vi "TaskFor_P3AT_Co_Boundary_Message.vi"(8 "error in (no error)":errorcluster caption="错误输入（无错误）", 10 "P3AT_Boundary":T1 {"max_rot" scale=0.0..1.0; "max_vel" scale=0.0..1.0}, 11 "Remote Endpoint P3AT输入":refnum<class "RemoteP3AT.lvclass">) -> (0 "error out":errorcluster caption="错误输出", 3 "Remote Endpoint P3AT输出":refnum<class "RemoteP3AT.lvclass">)   [LabVIEW 2014]
uses:
  RemoteP3AT.lvclass
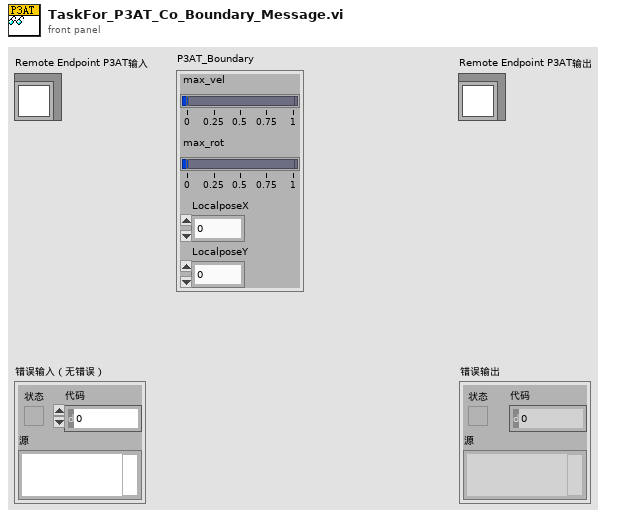
[diagram p1: front panel]
types:
  T1 = cluster{"max_vel":dbl, "max_rot":dbl, "LocalposeX":i32, "LocalposeY":i32}
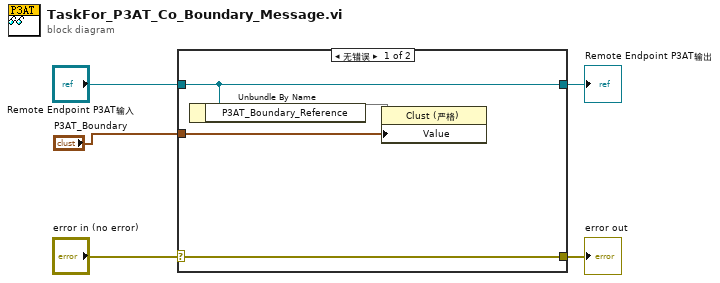
[diagram p0: block diagram]
diagram:
  n1 = case shown="无错误" "error in (no error)" {
    selector: "error in (no error)" -> [w9 w10]
    tunnel: [w9 w10] -> w4
    tunnel: [w8 w11] -> w2
    tunnel: "Remote Endpoint P3AT输入" -> [w8 w11]
    tunnel: "P3AT_Boundary" -> [w6 _]
    frame No Error {
      n2 = Unbundle By Name(w8) -> ("P3AT_Boundary_Reference"=w7)
      n3 = property class="Clust (严格)"(reference=w7, "Value"=w6) -> ()  [unwired: 1 in, 2 out]
    }
    frame Error {
    }
  }
  "error out" <- w4
  "Remote Endpoint P3AT输出" <- w2
